vi "Go At Angle.vi"(0 "Target Angle":dbl, 2 "Bot Angle":dbl=6.265957027809849, 3 "dt":dbl=0.03, 5 "Stop motors":bool, 6 "Speed":T1={"\nMoving speed"=1.0296610169491527, "Turning speed limit"=1.0169491525423728} {"Turning speed limit" scale=0.0..4.5; "Moving speed" scale=0.0..1.0}) -> ()   [LabVIEW 2017]
uses:
  Globals/Motor Speed Multiplier.vi
  <vilib>/addons/control/pid/pid.llb/PID (DBL).vi
  <vilib>/addons/control/pid/NI_PID_pid.lvlib
panel:
  in  "Turning PID":cluster{"P":dbl, "I":dbl, "D":dbl}={"P"=-0.8, "I"=0.0, "D"=0.007}
  in  "threshold angle":dbl=0.3
  out "Right motor speed":dbl=0.013786667806161291
  out "Left motor speed":dbl=-0.013786667806161291
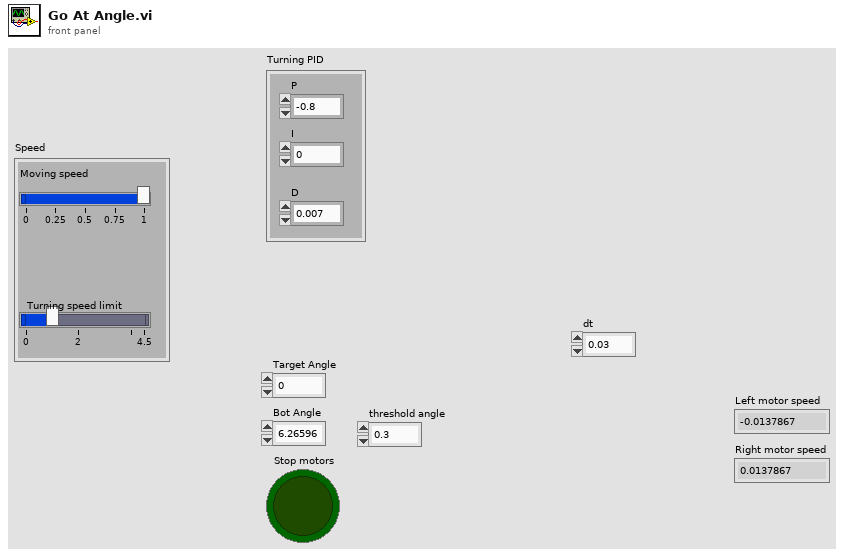
[diagram p1: front panel]
types:
  T1 = cluster{"\nMoving speed":dbl, "Turning speed limit":dbl}
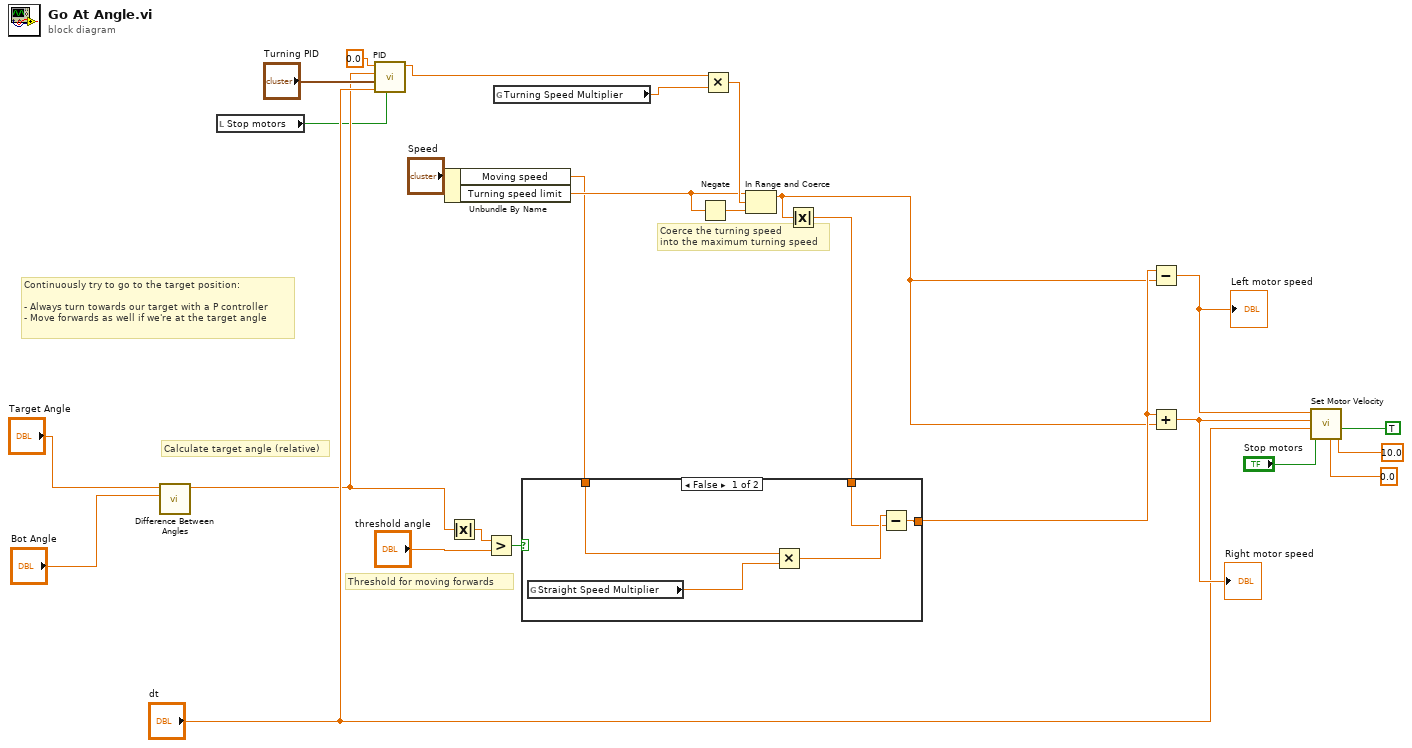
[diagram p0: block diagram]
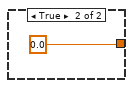
[diagram p2: hidden frame]
diagram:
  # "Coerce the turning speed\ninto the maximum turning speed"
  # "Threshold for moving forwards"
  # "Calculate target angle (relative)"
  # "Continuously try to go to the target position:\n\n- Always turn towards our target with a P controller\n- Move forwards as well if we're at the target angle"
  n1 = call "Difference Between Angles.vi"("Angle 2"="Bot Angle", "Angle 1"="Target Angle") -> ("Difference"=w9:dbl)  [unwired: 9 in]
  n2 = local read "Stop motors"() -> (w1:bool)
  n3 = call-poly <vilib>:"PID.vi"("reinitialize? (F)"=w1, "dt (s)"="dt", "PID gains"="Turning PID", "process variable"=w9, "setpoint"=0.0) -> ("output"=w5:dbl)  [unwired: 5 in, 1 out]
  n4 = Unbundle By Name("Speed") -> ("Moving speed"=w2:dbl, "Turning speed limit"=w6:dbl)
  n5 = Absolute Value(x=w9) -> (abs(x)=w21:dbl)
  n6 = Greater?(x=w21, y="threshold angle") -> (0:w17:bool)
  n7 = global read "Motor Speed Multiplier.vi" "Turning Speed Multiplier"() -> (w4:dbl)
  n8 = Negate(x=w6) -> (-x=w14:dbl)
  n9 = Multiply(x=w5, y=w4) -> (x*y=w15:dbl)
  n10 = In Range and Coerce(upper limit=w6, x=w15, lower limit=w14) -> (coerced(x)=w13:dbl)  [unwired: 1 out]
  n11 = Absolute Value(x=w13) -> (abs(x)=w12:dbl)
  n12 = case shown="False" w17 {
    tunnel: [w28 0.0] -> w18
    tunnel: w12 -> [w29 _]
    tunnel: w2 -> [w27 _]
    frame False {
      n13 = global read "Motor Speed Multiplier.vi" "Straight Speed Multiplier"() -> (w31:dbl)
      n14 = Multiply(x=w27, y=w31) -> (x*y=w30:dbl)
      n15 = Subtract(x=w30, y=w29) -> (x-y=w28:dbl)
    }
    frame True {
    }
  }
  n16 = Subtract(x=w18, y=w13) -> (x-y=w19:dbl)
  "Left motor speed" <- w19
  n17 = Add(x=w18, y=w13) -> (x+y=w20:dbl)
  "Right motor speed" <- w20
  n18 = call "Set Motor Velocity.vi"("Acceleration ramp constant"=10.0, "Accelerate?"=TRUE, "Back motor speed rev/s"=0.0 ("result"), "Disable motors"="Stop motors", "dt"="dt", "Right motor speed rev/s"=w20, "Left motor speed rev/s"=w19) -> ()  [unwired: 5 in]
